vi "Hausmodell.ReadZustandsgrössen.vi"(0 "Hausmodell in":refnum<data-value>, 5 "error in":errorcluster) -> (14 "Hausmodell out":refnum<data-value>, 16 "Raumtemperatur [°C]":dbl, 17 "Bodentemperatur [°C]":dbl, 18 "Rücklauftemperatur Heizkreislauf [°C]":dbl, 19 "error out":errorcluster)   [LabVIEW 2016, in "Hausmodell.lvclass"]
uses:
  Hausmodell.lvclass
  Hausmodell.lvclass/Hausmodell.ctl
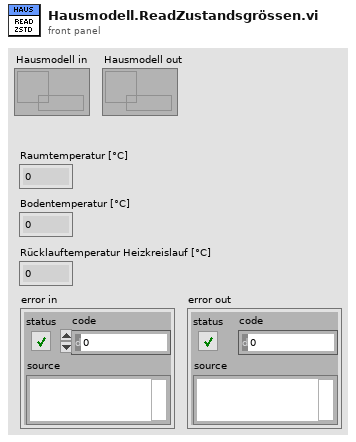
[diagram p1: front panel]
types:
  T1 = typedef "Hausmodell.lvclass/Hausmodell.Zustandsgrössen.ctl" = cluster{"Raumtemperatur [°C]":dbl, "Bodentemperatur [°C]":dbl, "Rücklauftemperatur Heizkreislauf [°C]":dbl}
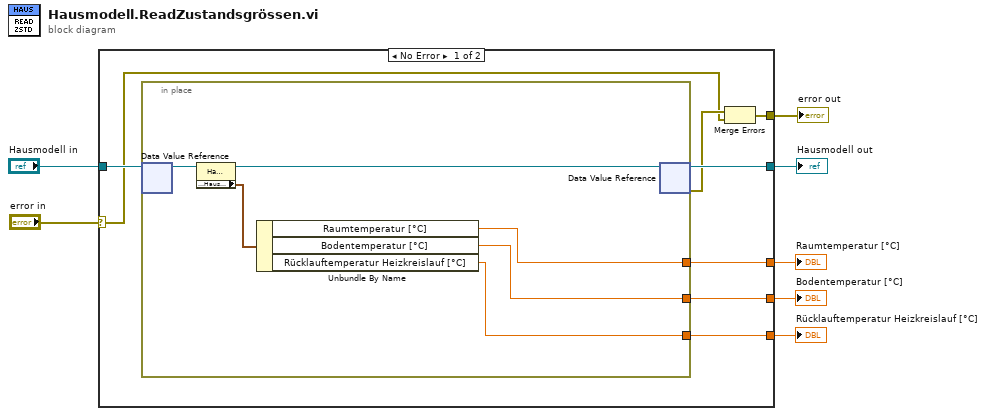
[diagram p0: block diagram]
diagram:
  n1 = case shown="No Error" "error in" {
    selector: "error in" -> [w8 w23]
    tunnel: "Hausmodell in" -> [w15 w22]
    tunnel: [w14 w22] -> w6
    tunnel: [w13 _] -> w5
    tunnel: [w12 _] -> w4
    tunnel: [w11 _] -> w3
    tunnel: [w10 w23] -> w1
    frame No Error {
      n2 = in-place {
        in-place-border: [w18] -> w13
        in-place-border: [w17] -> w12
        in-place-border: [w16] -> w11
        n3 = in-place-dvr #1(w15) -> (w21:refnum<class "Hausmodell.lvclass">)  [unwired: 1 out]
        n4 = property class="Hausmodell.lvclass"(reference=w21) -> (reference out=w20:refnum<class "Hausmodell.lvclass">, "Accessors:Zustandsgrössen.Hausmodell"=w19:T1)  [unwired: 1 in, 1 out]
        n5 = Unbundle By Name(w19) -> ("Raumtemperatur [°C]"=w18:dbl, "Bodentemperatur [°C]"=w17:dbl, "Rücklauftemperatur Heizkreislauf [°C]"=w16:dbl)
        n6 = in-place-dvr #1(w20) -> (w14:refnum<data-value>, w9:errorcluster)
      }
      n7 = Merge Errors(w9, w8) -> (w10:errorcluster)
    }
    frame Error {
    }
  }
  "Hausmodell out" <- w6
  "Raumtemperatur [°C]" <- w5
  "Bodentemperatur [°C]" <- w4
  "Rücklauftemperatur Heizkreislauf [°C]" <- w3
  "error out" <- w1
